vi "StrTo16.vi"(1 "StrIn":string) -> (0 "StrOut":string)   [LabVIEW 2013]
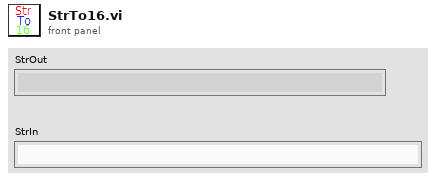
[diagram p1: front panel]
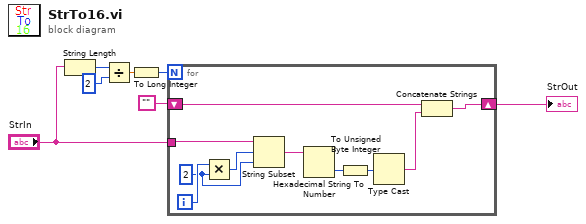
[diagram p0: block diagram]
diagram:
  n1 = String Length(string="StrIn") -> (length=w5:i32)
  n2 = Divide(x=w5, y=2) -> (x/y=w3:dbl)
  n3 = To Long Integer(number=w3) -> (32bit integer=w1:i32)
  n4 = for {
    N: w1 -> [_]
    tunnel: "StrIn" -> [w17]
    shift-right: [w10] -> w2
    shift-left: "" -> [w8]
    i -> [w16]
    w14 = 2 ("y")
    n5 = Multiply(x=w16, y=w14) -> (x*y=w15:i32)
    n6 = String Subset(string=w17, offset (0)=w15, length (rest)=w14) -> (substring=w13:string)
    n7 = Hexadecimal String To Number(string=w13) -> (number=w12:u32)  [unwired: 2 in, 1 out]
    n8 = To Unsigned Byte Integer(number=w12) -> (unsigned 8bit integer=w11:u8)
    n9 = Type Cast(x=w11) -> (*(type *) &x=w9:string)  [unwired: 1 in]
    n10 = Concatenate Strings(w8, w9) -> (w10:string)
  }
  "StrOut" <- w2
